vi "Read RN.vi"(10 "RN":i32, 11 "handle":i32) -> (1 "function return":i32, 2 "RN out":i32, 3 "handle out":i32)   [LabVIEW 2022 SP3]
doc: "BOOL H11890API __stdcall H11890ReadRN(HANDLE handle,DWORD *RN);"
uses:
  H11890api.dll
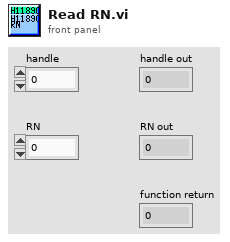
[diagram p1: front panel]
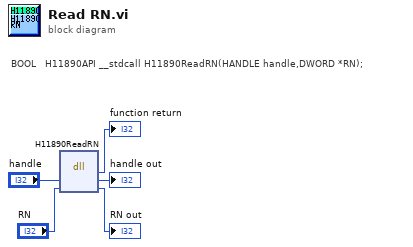
[diagram p0: block diagram]
diagram:
  # "BOOL\t\t\tH11890API __stdcall H11890ReadRN(HANDLE handle,DWORD *RN);"
  n1 = dll-call lib="C:/Users/Public/OneDrive/Desktop/PMT_Project_folder/PMT_VIs/H11890api.dll" fn="H11890ReadRN"("handle"="handle", "RN"="RN") -> ("Return"=→"function return":i32, "handle"=→"handle out":i32, "RN"=→"RN out":i32)  [unwired: 3 in, 2 out]
